vi "Extract frequence et puissance.vi"(9 "Frequence Stop":dbl=435.5 format="%#_13g", 10 "Frequence Start":dbl=430.5 format="%#_13g", 11 "Reception RSA306":string) -> (2 "DBMax":dbl, 3 "Freq":dbl format="%#.6f")   [LabVIEW 2020, in "Library Instrument & Equipement.lvlib" / "Library Spectrum Analyser.lvlib" / "Class Spectrum_Analyser RS306B.lvclass"]
uses:
  Class Spectrum_Analyser RS306B.lvclass
  Class Spectrum_Analyser RS306B.lvclass/Class Spectrum_Analyser RS306B.ctl
panel:
  out "Freq 2":dbl format="%#.6f"
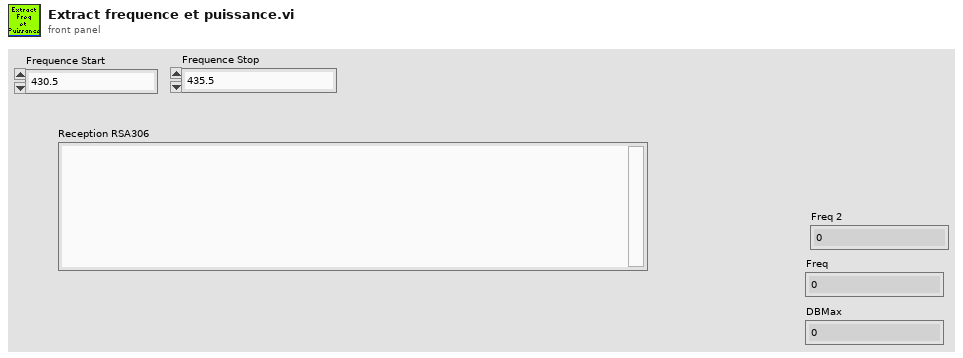
[diagram p1: front panel]
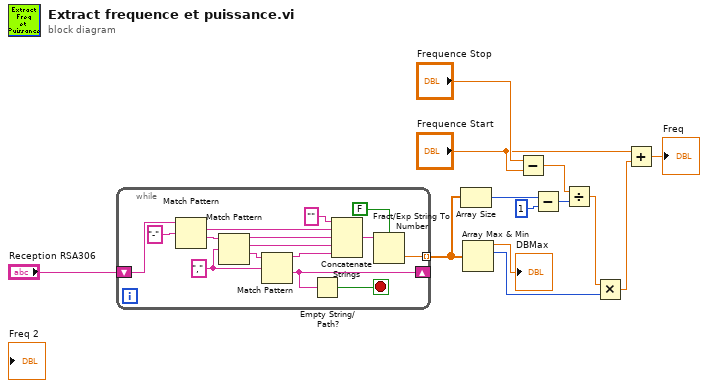
[diagram p0: block diagram]
diagram:
  n1 = while {
    shift-right: [w18] -> _
    shift-left: "Reception RSA306" -> [w28]
    tunnel: [w15] -> w10 mode=indexing
    stop <- w17 stop-if-true
    w20 = "," ("expression régulière")
    n2 = Match Pattern(string=w28, regular expression="-" ("expression régulière")) -> (match substring=w26:string, after substring=w24:string)  [unwired: 1 in, 2 out]
    n3 = Match Pattern(string=w24, regular expression=w20) -> (before substring=w23:string, match substring=w22:string, after substring=w21:string)  [unwired: 1 in, 1 out]
    n4 = Match Pattern(string=w21, regular expression=w20) -> (before substring=w19:string, after substring=w18:string)  [unwired: 1 in, 2 out]
    n5 = Empty String/Path?(string/path=w18) -> (empty?=w17:bool)
    n6 = Concatenate Strings("" ("expression régulière"), w26, w23, w22, w19) -> (w16:string)
    n7 = Fract/Exp String To Number(use system decimal point (T)=FALSE ("utiliser le séparateur décimal du système (V)"), string=w16) -> (number=w15:dbl)  [unwired: 2 in, 1 out]
  }
  n8 = Array Size(array=w10) -> (size(s)=w3:i32)
  n9 = Array Max & Min(array=w10) -> (max value=→"DBMax":dbl, max index (indices)=w9:i32)  [unwired: 2 out]
  n10 = Subtract(x="Frequence Stop", y="Frequence Start") -> (x-y=w11:dbl)
  n11 = Subtract(x=w3, y=1) -> (x-y=w1:i32)
  n12 = Divide(x=w11, y=w1) -> (x/y=w8:dbl)
  n13 = Multiply(x=w8, y=w9) -> (x*y=w7:dbl)
  n14 = Add(x="Frequence Start", y=w7) -> (x+y=→"Freq":dbl)
